vi "Create BBOX Data (SubVI).vi"(10 "Left":u16=150, 11 "Top":u16) -> (3 "BBOX Point":u64)   [LabVIEW 2015]
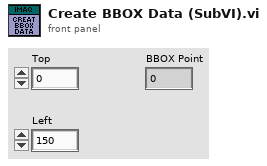
[diagram p1: front panel]
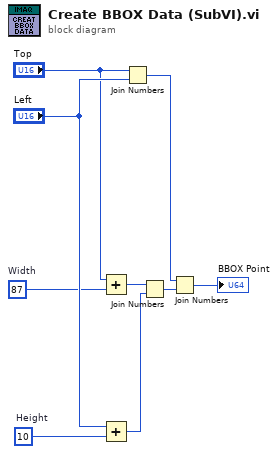
[diagram p0: block diagram]
diagram:
  w2 = u16 10  # Height
  w1 = u16 87  # Width
  n1 = Add(x="Top", y=w1) -> (x+y=w6:u16)
  n2 = Add(x="Left", y=w2) -> (x+y=w7:u16)
  n3 = Join Numbers(hi="Top", lo="Left") -> ((hi.lo)=w3:u32)
  n4 = Join Numbers(hi=w6, lo=w7) -> ((hi.lo)=w4:u32)
  n5 = Join Numbers(hi=w3, lo=w4) -> ((hi.lo)=→"BBOX Point":u64)
